vi "HFRR ADV v031 new software.vi"() -> ()   [LabVIEW 2025] (continued)
                        n2406 = Concatenate Strings("Applied Load [grams] :" ("Content"), w3458) -> (w3460:string)
                        n2407 = local read "EVENT LOG"() -> (w3462:string)
                        n2408 = call "Event Log.vi"("Content"=w3460, "EVENT LOG"=w3462) -> ("EVENT LOG"=w3461:string)  [unwired: 8 in, 1 out]
                        n2409 = local write "EVENT LOG"(w3461) -> ()
                      }
                      frame #24 {
                        n2410 = Wait (ms)(milliseconds to wait=u32 50) -> ()  [unwired: 1 out]
                      }
                      frame #25 {
                        n2411 = local read "Set Strk"() -> (w3465:dbl)
                        n2412 = Number To Fractional String(number=w3465, precision (6)=i16 2) -> (F-format string=w3466:string)  [unwired: 2 in]
                        n2413 = Concatenate Strings("Set Stroke [mm] :" ("Content"), w3466) -> (w3468:string)
                        n2414 = local read "EVENT LOG"() -> (w3470:string)
                        n2415 = call "Event Log.vi"("Content"=w3468, "EVENT LOG"=w3470) -> ("EVENT LOG"=w3469:string)  [unwired: 8 in, 1 out]
                        n2416 = local write "EVENT LOG"(w3469) -> ()
                      }
                      frame #26 {
                        n2417 = Wait (ms)(milliseconds to wait=u32 50) -> ()  [unwired: 1 out]
                      }
                      frame #27 {
                        n2418 = local read "Set Temp"() -> (w3473:dbl)
                        n2419 = Number To Fractional String(number=w3473, precision (6)=i16 2) -> (F-format string=w3474:string)  [unwired: 2 in]
                        n2420 = Concatenate Strings("Set Temperature [deg C] :" ("Content"), w3474) -> (w3476:string)
                        n2421 = local read "EVENT LOG"() -> (w3478:string)
                        n2422 = call "Event Log.vi"("Content"=w3476, "EVENT LOG"=w3478) -> ("EVENT LOG"=w3477:string)  [unwired: 8 in, 1 out]
                        n2423 = local write "EVENT LOG"(w3477) -> ()
                      }
                      frame #28 {
                        n2424 = Wait (ms)(milliseconds to wait=u32 50) -> ()  [unwired: 1 out]
                      }
                      frame #29 {
                        n2425 = local read "Set Rh"() -> (w3481:dbl)
                        n2426 = Number To Fractional String(number=w3481, precision (6)=i16 2) -> (F-format string=w3482:string)  [unwired: 2 in]
                        n2427 = Concatenate Strings("Set Humidity [%RH] :" ("Content"), w3482) -> (w3484:string)
                        n2428 = local read "EVENT LOG"() -> (w3486:string)
                        n2429 = call "Event Log.vi"("Content"=w3484, "EVENT LOG"=w3486) -> ("EVENT LOG"=w3485:string)  [unwired: 8 in, 1 out]
                        n2430 = local write "EVENT LOG"(w3485) -> ()
                      }
                      frame #30 {
                        n2431 = Wait (ms)(milliseconds to wait=u32 50) -> ()  [unwired: 1 out]
                      }
                      frame #31 {
                        n2432 = local read "test time"() -> (w3489:dbl)
                        n2433 = Number To Fractional String(number=w3489, precision (6)=i16 1) -> (F-format string=w3490:string)  [unwired: 2 in]
                        n2434 = Concatenate Strings("Test Duration [mins] :" ("Content"), w3490) -> (w3492:string)
                        n2435 = local read "EVENT LOG"() -> (w3494:string)
                        n2436 = call "Event Log.vi"("Content"=w3492, "EVENT LOG"=w3494) -> ("EVENT LOG"=w3493:string)  [unwired: 8 in, 1 out]
                        n2437 = local write "EVENT LOG"(w3493) -> ()
                      }
                      frame #32 {
                        w3495 = dbl[] [] ("History Data")
                        w3496 = cluster{"y":dbl, dbl, "y":dbl}[] [] ("History Data")
                        w3497 = FALSE ("Visible")
                        n2438 = property on="Stroke ( mm )" class="WFChart (strict)"("History Data"=w3496) -> ()  [unwired: 2 in, 2 out]
                        n2439 = property on="Humidity ( %RH )" class="WFChart (strict)"("History Data"=w3495) -> ()  [unwired: 2 in, 2 out]
                        n2440 = property on="Temperature ( Deg C )" class="WFChart (strict)"("History Data"=w3495) -> ()  [unwired: 2 in, 2 out]
                        n2441 = property on="Electrical Contact Resistance ( % )" class="WFChart (strict)"("History Data"=w3495) -> ()  [unwired: 2 in, 2 out]
                        n2442 = property on="Coefficient of Friction" class="WFChart (strict)"("History Data"=w3495) -> ()  [unwired: 2 in, 2 out]
                        n2443 = property on="Frictional Force ( N )" class="WFChart (strict)"("History Data"=w3495) -> ()  [unwired: 2 in, 2 out]
                        n2444 = property on="Coefficient of Friction" class="WFChart (strict)"("History Data"=w3495) -> ()  [unwired: 2 in, 2 out]
                        n2445 = property on="Frictional Force ( N )" class="WFChart (strict)"("History Data"=w3495) -> ()  [unwired: 2 in, 2 out]
                        n2446 = property on="Electrical Contact Resistance ( % )" class="WFChart (strict)"("History Data"=w3495) -> ()  [unwired: 2 in, 2 out]
                        n2447 = property on="Humidity ( %RH )" class="WFChart (strict)"("History Data"=w3495) -> ()  [unwired: 2 in, 2 out]
                        n2448 = property on="Stroke ( mm )" class="WFChart (strict)"("History Data"=w3496) -> ()  [unwired: 2 in, 2 out]
                        n2449 = property on="Temperature ( Deg C )" class="WFChart (strict)"("History Data"=w3495) -> ()  [unwired: 2 in, 2 out]
                        n2450 = property on="Service Password Log" class="Str"("Visible"=w3497) -> ()  [unwired: 2 in, 2 out]
                        n2451 = property on="Password 3" class="Clust (strict)"("Visible"=w3497) -> ()  [unwired: 2 in, 2 out]
                      }
                    }
                    "TEST FILE NAM,E SAVED" <- TRUE ("TEST FILE NAM,E SAVED")
                  }
                }
              }
            }
          }
        }
        n2452 = local write "Test \nStatus"(w2886) -> ()
        n2453 = local write "Save"(w2886) -> ()
        n2454 = local read "Main Tab"() -> (w2880:T2)
        n2455 = case shown="True" w2883 {
          frame False {
            n2456 = local read "Rt 3"() -> (w2955:bool)
            n2457 = case shown="True" w2955 {
              frame False {
              }
              frame True {
                n2458 = local write "Rt 3"(FALSE ("Rt 3")) -> ()
              }
            }
            "Rt" <- TRUE ("Rt")
            "Rt 2" <- FALSE ("Rt")
          }
          frame True {
            n2459 = local read "Rt"() -> (w2961:bool)
            n2460 = local write "Rt 2"(TRUE ("Rt 2")) -> ()
            n2461 = case shown="True" w2961 {
              frame False {
              }
              frame True {
                n2462 = local write "Rt"(FALSE ("Rt")) -> ()
              }
            }
            "Rt 3" <- TRUE ("Rt 3")
          }
        }
        n2463 = case shown="\"Acquire\"" w2880 {
          tunnel: w2882 -> [_ w2989]
          frame Default {
            w2988 = 0.0 ("output")
            n2464 = local write "PID-out"(w2988) -> ()
            n2465 = local write "Frequency ( Hz )"(w2988) -> ()
          }
          frame "Acquire" {
            n2466 = stacked-sequence {
              frame #0 {
                n2467 = local read "Auto Start Test"() -> (w2991:bool)
                n2468 = case shown="True" w2991 {
                  tunnel: "RUN" -> [w3012 w3015]
                  tunnel: [w3012 w3014] -> w2992
                  frame False {
                  }
                  frame True {
                    n2469 = local read "Auto Start Temp"() -> (w3013:bool)
                    n2470 = Or(x=w3015, y=w3013) -> (x .or. y?=w3014:bool)
                  }
                }
                n2471 = local read "clk"() -> (w3011:dbl)
                n2472 = local read "Save"() -> (w3007:bool)
                n2473 = Equal?(x=w3011, y=0.0) -> (x = y?=w3008:bool)
                n2474 = And(x=w3008, y=w3007) -> (x .and. y?=w3009:bool)
                n2475 = Not(x="Engage") -> (.not. x?=w2998:bool)
                n2476 = case shown="False" w2992 {
                  tunnel: [0.0 w3038] -> w2994
                  frame False {
                    (unwired) TRUE ("Visible")
                    n2477 = local read "Auto Start Test"() -> (w3019:bool)
                    n2478 = local write "Start Time"(TRUE ("Start Time")) -> ()
                    n2479 = property on="Stroke 2" class="DigNum (strict)"("Visible"=FALSE) -> ()  [unwired: 2 in, 2 out]
                    n2480 = case shown="False" w3019 {
                      frame False {
                        n2481 = property on="Heater Button" class="Bool (strict)"("DisabledEnum"=T19."Enabled" ("Disabled")) -> ()  [unwired: 2 in, 2 out]
                        n2482 = property on="Humidity" class="Bool (strict)"("DisabledEnum"=T19."Enabled" ("Disabled")) -> ()  [unwired: 2 in, 2 out]
                      }
                      frame True {
                      }
                    }
                    n2483 = case shown="False" "TestCompFlg" {
                      frame False {
                        n2484 = local read "StartFlg"() -> (w3027:bool)
                        n2485 = case shown="True" w3027 {
                          frame False {
                          }
                          frame True {
                            n2486 = stacked-sequence {
                              frame #0 {
                                n2487 = local read "EVENT LOG"() -> (w3031:string)
                                n2488 = call "Event Log.vi"("Content"="Test was interrupted", "EVENT LOG"=w3031) -> ("EVENT LOG"=w3032:string)  [unwired: 8 in, 1 out]
                                n2489 = local write "EVENT LOG"(w3032) -> ()
                                n2490 = property on="RUN" class="Bool (strict)"("Visible"=TRUE) -> ()  [unwired: 2 in, 2 out]
                                n2491 = property on="Auto Start Test" class="Bool (strict)"("Visible"=TRUE) -> ()  [unwired: 2 in, 2 out]
                              }
                              frame #1 {
                                w3034 = FALSE ("StartFlg")
                                n2492 = property on="Heater Button" class="Bool (strict)"("Val(Sgnl)"=FALSE ("Value (Signaling)")) -> ()  [unwired: 2 in, 2 out]
                                n2493 = local write "Heater Button"(w3034) -> ()
                                n2494 = local write "StartFlg"(w3034) -> ()
                                n2495 = local write "Humidity"(w3034) -> ()
                              }
                              frame #2 {
                                n2496 = local write "Due Write"("VC;0" ("Command")) -> ()
                              }
                              frame #3 {
                                n2497 = Wait (ms)(milliseconds to wait=u32 1500) -> ()  [unwired: 1 out]
                              }
                              frame #4 {
                                n2498 = local write "Due Write"("HE;0" ("Command")) -> ()
                              }
                            }
                          }
                        }
                      }
                      frame True {
                      }
                    }
                    n2499 = local write "String 14"("Test will autostart once parameters reach the set value." ("String 14")) -> ()
                  }
                  frame True {
                    (unwired) FALSE ("Visible")
                    n2500 = property on="Stroke 2" class="DigNum (strict)"("Visible"=TRUE) -> ()  [unwired: 2 in, 2 out]
                    n2501 = property on="STOP 2" class="Bool (strict)"("Disabled"=u8 2) -> ()  [unwired: 2 in, 2 out]
                    n2502 = local write "String 14"(" Running....." ("String 14")) -> ()
                    n2503 = property on="Heater Button" class="Bool (strict)"("DisabledEnum"=T19."Disabled and Grayed Out" ("Disabled")) -> ()  [unwired: 2 in, 2 out]
                    n2504 = property on="Humidity" class="Bool (strict)"("DisabledEnum"=T19."Disabled and Grayed Out" ("Disabled")) -> ()  [unwired: 2 in, 2 out]
                    n2505 = case shown="True" "Start Time" {
                      selector: "Start Time" -> [_ w3057]
                      frame False {
                      }
                      frame True {
                        n2506 = Not(x=w3057) -> (.not. x?=w3056:bool)
                        n2507 = local write "Start Time"(w3056) -> ()
                        n2508 = local read "EVENT LOG"() -> (w3058:string)
                        n2509 = call "Event Log.vi"("Content"="Test in progress", "EVENT LOG"=w3058) -> ("EVENT LOG"=w3060:string)  [unwired: 8 in, 1 out]
                        n2510 = local write "EVENT LOG"(w3060) -> ()
                      }
                    }
                    n2511 = disable-structure shown="Enabled" {
                      disable-tunnel: [w3049 w3055] -> w3038
                      frame Disabled {
                        n2512 = local read "Set Hz"() -> (w3052:dbl)
                        n2513 = call <vilib>:"Uniform White Noise Waveform.vi"() -> ("signal out"=w3051:waveform(dbl))  [unwired: 10 in, 1 out]
                        n2514 = Random Number (0-1)() -> (number: 0 to 1=w3048:dbl)
                        n2515 = Add(x=w3052, y=w3051) -> (x+y=w3050:waveform(dbl))
                        n2516 = Multiply(x=ext 0.01 ("y"), y=w3048) -> (x*y=w3046:ext)
                        n2517 = Multiply(x=w3050, y=w3046) -> (x*y=w3049:waveform(ext))
                      }
                      frame Enabled {
                        n2518 = call-poly <vilib>:"Random Number (Range).vi"("lower bound (0)"=49.89, "upper bound (100)"=50.8) -> ("number"=w3055:dbl)  [unwired: 9 in]
                      }
                    }
                    "StartFlg" <- TRUE ("StartFlg")
                  }
                }
                n2519 = case shown="True" w3009 {
                  frame False {
                  }
                  frame True {
                    n2520 = local write "clk"(10.0 ("clk")) -> ()
                    n2521 = Get Date/Time In Seconds() -> (seconds since 1Jan1904=w3063:timestamp)
                    n2522 = To Double Precision Float(number=w3063) -> (double precision float=w3061:dbl)
                    n2523 = local write "acq timer"(w3061) -> ()
                    n2524 = local write "act save time"(w3061) -> ()
                  }
                }
                n2525 = call "Elapsed Time"("Time Target (s)"="Countdown", "Reset"=w2998) -> ("Elapsed Time (s)"=w3003:dbl, "Time has Elapsed"=w3001:bool)  [unwired: 10 in, 6 out]
                "Countdown 2" <- w3003
                n2526 = Subtract(x=w3003, y=2.0) -> (x-y=w3006:dbl)
                n2527 = Less?(x=w3006, y="Countdown") -> (x < y?=w3004:bool)
                n2528 = And(x=w3004, y=w3001) -> (x .and. y?=w3000:bool)
                n2529 = case shown="True" w3000 {
                  frame False {
                  }
                  frame True {
                    (unwired) dbl[] [] ("History Data")
                    n2530 = local write "Engage"(FALSE ("Engage")) -> ()
                    n2531 = local write "RUN"(TRUE ("RUN")) -> ()
                    n2532 = local read "Humidity ( %RH )"() -> (→"Rh Before":dbl)
                  }
                }
                n2533 = local read "Test \nStatus"() -> (w2996:bool)
                n2534 = Select(t=w2994, s=w2996, f=0.0) -> (s? t:f=w2995:dbl)
                n2535 = local write "Frequency ( Hz )"(w2995) -> ()
              }
              frame #1 {
                w3086 = 1000000.0 ("x")
                # "HC;1/0\nST;VALUE"
                # "Elapsed time\ncof\nstroke\nAir temp\nTemp\nHumidity"
                # "acq timer\n\nact save time"
                # "convert to microseconds"
                n2536 = local read "COUNT"() -> (w3069:i32)
                n2537 = local read "Rate"() -> (w3082:dbl)
                n2538 = Divide(x=w3086, y=w3082) -> (x/y=w3087:dbl)
                n2539 = Greater Or Equal?(x=w3069, y=250) -> (x >= y?=w3068:bool)
                n2540 = Get Date/Time In Seconds() -> (seconds since 1Jan1904=w3089:timestamp)
                n2541 = case shown="True" w3068 {
                  frame False {
                    n2542 = local read "COUNT"() -> (w3090:i32)
                    n2543 = Increment(x=w3090) -> (x+1=w3091:i32)
                    n2544 = local write "COUNT"(w3091) -> ()
                  }
                  frame True {
                    n2545 = local write "COUNT"(0 ("COUNT")) -> ()
                  }
                }
                n2546 = local read "Samplingtime 2"() -> (w3067:dbl)
                n2547 = local read "act save time"() -> (w3084:dbl)
                n2548 = Divide(x=w3087, y=w3086) -> (x/y=w3085:dbl)
                n2549 = To Double Precision Float(number=w3089) -> (double precision float=w3078:dbl)
                n2550 = Add(x=w3084, y=w3067) -> (x+y=w3083:dbl)
                n2551 = local read "acq timer"() -> (w3088:dbl)
                n2552 = local read "COUNT"() -> (w3071:i32)
                n2553 = Greater Or Equal?(x=w3078, y=w3083) -> (x >= y?=w3066:bool)
                n2554 = Multiply(x=w3085, y=w3071) -> (x*y=w3077:dbl)
                n2555 = Subtract(x=w3078, y=w3088) -> (x-y=w3080:dbl)
                n2556 = local read "Save"() -> (w3081:bool)
                n2557 = Add(x=w3080, y=w3077) -> (x+y=w3064:dbl)
                "Elapsed time 3" <- w3064
                n2558 = And(x=w3066, y=w3081) -> (x .and. y?=w3079:bool)
                n2559 = Divide(x=w3064, y=60.0) -> (x/y=w3075:dbl)
                n2560 = local read "Test \nStatus"() -> (w3065:bool)
                n2561 = local read "clk"() -> (w3072:dbl)
                n2562 = Equal?(x=w3072, y=10.0) -> (x = y?=w3074:bool)
                n2563 = case shown="True" w3079 {
                  tunnel: w3078 -> [_ w3203]
                  tunnel: [FALSE ("Boolean 2") TRUE ("Boolean 2")] -> _
                  frame False {
                  }
                  frame True {
                    w3157 = ";" ("Substring")
                    # "Pid out/\nFreq response value"
                    n2564 = local write "act save time"(w3203) -> ()
                    n2565 = local read "FILE"() -> (w3151:string)
                    n2566 = call "file check.vi"("file name in"=w3151) -> ("error out"=w3154:errorcluster, "file name out"=w3149:string)  [unwired: 9 in]
                    n2567 = local read "LVDT STROKE"() -> (w3146:dbl)
                    n2568 = local read "Add up Stroke"() -> (w3144:dbl)
                    n2569 = call "FILE PATH CREATION.vi"("error in"=w3154, "FILE NAME :"=w3149) -> ("FILE OUT"=w3152:path)  [unwired: 8 in, 1 out]
                    n2570 = Concatenate Strings(w3149, ".dgf" ("Substring")) -> (w3153:string)
                    n2571 = Subtract(x=w3146, y=w3144) -> (x-y=w3145:dbl)
                    n2572 = Absolute Value(x=w3145) -> (abs(x)=w3143:dbl)
                    n2573 = local read "FF 2"() -> (→"Frictional Force ( N )" →"Frictional Force ( N )":dbl)
                    n2574 = Build Path(base path=w3152, name or relative path=w3153) -> (appended path=w3148:path)
                    n2575 = local read "COF 2"() -> (w3162:dbl)
                    "Coefficient of Friction" <- w3162
                    "COF 4" <- w3162
                    "Coefficient of Friction" <- w3162
                    n2576 = local read "TEMP"() -> (w3165:dbl)
                    "Temperature ( Deg C )" <- w3165
                    n2577 = local read "Humidity ( %RH )"() -> (w3164:dbl)
                    "Humidity ( %RH )" <- w3164
                    "Humidity ( %RH )" <- w3164
                    n2578 = local read "Frequency ( Hz )"() -> (w3171:dbl)
                    n2579 = local read "LVDT STROKE DISPLAY"() -> (w3140:dbl)
                    n2580 = call <vilib>:"Mean PtByPt.vi"("x"=w3143, "sample length"="STROKE FILTER") -> ("mean"=→"LVDT STROKE Actual":dbl)  [unwired: 2 in, 1 out]
                    n2581 = local read "Elapsed time"() -> (w3196:dbl)
                    n2582 = local read "AIR TEMP"() -> (w3169:dbl)
                    n2583 = local read "PID-out"() -> (w3174:dbl)
                    n2584 = local write "Temperature ( Deg C )"(w3165) -> ()
                    n2585 = Number To Fractional String(number=w3140, width (-)=i16 9 ("precision (6)"), precision (6)=i16 6) -> (F-format string=w3189:string)  [unwired: 1 in]
                    n2586 = Number To Fractional String(number=w3169, width (-)=i16 9 ("precision (6)"), precision (6)=i16 3) -> (F-format string=w3188:string)  [unwired: 1 in]
                    n2587 = Number To Fractional String(number=w3165, width (-)=i16 9 ("precision (6)"), precision (6)=i16 3) -> (F-format string=w3185:string)  [unwired: 1 in]
                    n2588 = Number To Fractional String(number=w3164, width (-)=i16 9 ("precision (6)"), precision (6)=i16 3) -> (F-format string=w3182:string)  [unwired: 1 in]
                    n2589 = Number To Fractional String(number=0.0, width (-)=i16 9 ("precision (6)"), precision (6)=i16 3) -> (F-format string=w3179:string)  [unwired: 1 in]
                    n2590 = Number To Fractional String(number=w3174, width (-)=i16 9 ("precision (6)"), precision (6)=i16 3) -> (F-format string=w3175:string)  [unwired: 1 in]
                    n2591 = Number To Fractional String(number=w3171, width (-)=i16 9 ("precision (6)"), precision (6)=i16 3) -> (F-format string=w3170:string)  [unwired: 1 in]
                    n2592 = Number To Fractional String(number=w3162, width (-)=i16 9 ("precision (6)"), precision (6)=i16 6) -> (F-format string=w3197:string)  [unwired: 1 in]
                    n2593 = Number To Fractional String(number=w3196, width (-)=i16 14 ("precision (6)"), precision (6)=i16 3) -> (F-format string=w3198:string)  [unwired: 1 in]
                    n2594 = Bundle("y"=1.02, "LVDT STROKE DISPLAY"=w3140, "y"=0.98) -> (w3163:T30)  [unwired: 1 in]
                    n2595 = Number To Fractional String(number="Ambient Humidity :", width (-)=i16 9 ("precision (6)"), precision (6)=i16 6) -> (F-format string=w3155:string)  [unwired: 1 in]
                    n2596 = local read "RUN"() -> (w3161:bool)
                    n2597 = case shown="True" w3161 {
                      tunnel: w3163 -> [_ w3208]
                      tunnel: w3140 -> [_ w3207]
                      tunnel: w3140 -> [_ w3205]
                      tunnel: w3140 -> [_ w3206]
                      frame False {
                      }
                      frame True {
                        "Stroke ( mm )" <- w3208
                        "Stroke ( mm )" <- w3208
                        "Stroke 4" <- w3207
                        "Stroke 3" <- w3205
                        "Stroke 2" <- w3206
                        "measured_stroke" <- w3205
                      }
                    }
                    n2598 = Concatenate Strings(w3198, w3157, w3197, w3157, w3189, w3157, w3188, w3157, w3185, w3157, w3182, w3157, w3179, w3157, w3175, w3157, w3170, w3157, w3155, "\r") -> (w3195:string)
                    n2599 = call <vilib>:"Write Characters To File.vi"("append to file? (new file:F)"=TRUE, "character string"=w3195, "file path (dialog if empty)"=w3148) -> ()  [unwired: 2 in, 1 out]
                    "refresh flag" <- TRUE ("refresh flag")
                  }
                }
                n2600 = case shown="True" w3065 {
                  tunnel: w3075 -> [_ w3101]
                  tunnel: w3080 -> [_ w3111]
                  tunnel: [0.0 w3107] -> _
                  tunnel: w3074 -> [_ w3106]
                  tunnel: [0.0 w3105] -> _
                  tunnel: w3064 -> [_ w3105]
                  tunnel: w3078 -> [w3094 _]
                  frame False {
                    n2601 = local write "acq timer"(w3094) -> ()
                    n2602 = local write "Test Duration Status"(0.0 ("Test Duration Status")) -> ()
                  }
                  frame True {
                    n2603 = local read "Set Hz"() -> (w3108:dbl)
                    n2604 = local write "Elapsed time"(w3101) -> ()
                    n2605 = local read "test time"() -> (w3100:dbl)
                    n2606 = Multiply(x=w3111, y=w3108) -> (x*y=w3110:dbl)
                    n2607 = case shown="False" w3106 {
                      tunnel: w3110 -> [w3112 _]
                      tunnel: [w3112 1.0] -> w3107
                      frame False {
                        n2608 = local write "Cycles elapsed"(w3112) -> ()
                      }
                      frame True {
                      }
                    }
                    n2609 = Greater?(x=w3101, y=w3100) -> (0:w3109:bool)
                    n2610 = Subtract(x=w3100, y=w3101) -> (x-y=w3099:dbl)
                    n2611 = Multiply(x=w3099, y=60.0) -> (x*y=w3098:dbl)
                    n2612 = local write "Time Remaining"(w3098) -> ()
                    n2613 = local write "Remaining Time"(w3098) -> ()
                    n2614 = case shown="True" w3109 {
                      frame False {
                      }
                      frame True {
                        n2615 = stacked-sequence {
                          frame #0 {
                            w3117 = T19."Enabled" ("Disabled")
                            w3116 = FALSE ("TEST FILE NAM,E SAVED")
                            w3118 = "" ("FILE")
                            w3119 = TRUE ("Visible")
                            n2616 = local write "Humidity"(FALSE ("Humidity")) -> ()
                            n2617 = local write "RUN"(FALSE ("OK Button 2")) -> ()
                            n2618 = local write "Heater Button"(FALSE ("Heater Button")) -> ()
                            n2619 = local write "Auto Start Test"(FALSE ("Auto Start Test")) -> ()
                            n2620 = local write "TestCompFlg"(TRUE ("StpFlg")) -> ()
                            n2621 = local read "Humidity ( %RH )"() -> (→"Rh After":dbl)
                            n2622 = property on="STOP 2" class="Bool (strict)"("Disabled"=u8 0) -> ()  [unwired: 2 in, 2 out]
                            n2623 = local read "EVENT LOG"() -> (w3124:string)
                            n2624 = call "Event Log.vi"("Content"="Test Completed", "EVENT LOG"=w3124) -> ("EVENT LOG"=w3123:string)  [unwired: 8 in, 1 out]
                            n2625 = property on="RUN" class="Bool (strict)"("Visible"=w3119) -> ()  [unwired: 2 in, 2 out]
                            n2626 = property on="Auto Start Test" class="Bool (strict)"("Visible"=w3119) -> ()  [unwired: 2 in, 2 out]
                            n2627 = local write "Batch Ref Num :"(w3118) -> ()
                            n2628 = local write "FILE"(w3118) -> ()
                            n2629 = local write "EVENT LOG"(w3123) -> ()
                            n2630 = local write "TEST FILE NAM,E SAVED"(w3116) -> ()
                            n2631 = local write "Fuel Discription :"(w3118) -> ()
                            n2632 = local write "START TEMP"(w3116) -> ()
                            n2633 = local write "Remarks :"(w3118) -> ()
                            n2634 = local write "Main Dashboard Buttons"(T1."Imaging" ("Main Dashboard Buttons")) -> ()
                            n2635 = local write "Main Tab"(T2."Adv Scar" ("Main Tab")) -> ()
                            n2636 = property on="FRICVALZ 2" class="Bool (strict)"("DisabledEnum"=w3117) -> ()  [unwired: 2 in, 2 out]
                            n2637 = property on="FRICVALZ 3" class="Bool (strict)"("DisabledEnum"=w3117) -> ()  [unwired: 2 in, 2 out]
                            n2638 = property on="FRICVALZ 4" class="Bool (strict)"("DisabledEnum"=w3117) -> ()  [unwired: 2 in, 2 out]
                          }
                          frame #1 {
                            n2639 = Wait (ms)(milliseconds to wait=u32 1500) -> ()  [unwired: 1 out]
                          }
                          frame #2 {
                            n2640 = local write "Due Write"("VC;0") -> ()
                          }
                          frame #3 {
                            n2641 = Wait (ms)(milliseconds to wait=u32 1500) -> ()  [unwired: 1 out]
                          }
                          frame #4 {
                            n2642 = local write "Due Write"("VC;0") -> ()
                          }
                          frame #5 {
                            n2643 = Wait (ms)(milliseconds to wait=u32 1500) -> ()  [unwired: 1 out]
                          }
                          frame #6 {
                            n2644 = local write "Due Write"("ST;0") -> ()
                          }
                          frame #7 {
                            n2645 = local write "measured_stroke"(0.0 ("measured_stroke")) -> ()
                            n2646 = Wait (ms)(milliseconds to wait=u32 1500) -> ()  [unwired: 1 out]
                          }
                          frame #8 {
                            n2647 = local write "Due Write"("HE;0") -> ()
                          }
                        }
                      }
                    }
                    n2648 = Divide(x=w3101, y=w3100) -> (x/y=w3104:dbl)
                    n2649 = Multiply(x=w3104, y=100.0) -> (x*y=w3102:dbl)
                    n2650 = local write "Test Duration Status"(w3102) -> ()
                  }
                }
              }
              frame #2 {
                n2651 = case shown="True" "Heater Button" {
                  tunnel: [0.0 ("output") w3231] -> w3209
                  frame False {
                    w3212 = TRUE ("tmpchk")
                    n2652 = local read "TEMP"() -> (w3213:dbl)
                    n2653 = local write "Temp ini"(w3213) -> ()
                    n2654 = local write "Reset 4"(w3212) -> ()
                    n2655 = local write "tmpchk"(w3212) -> ()
                    n2656 = local write "reinit"(TRUE ("reinit")) -> ()
                    n2657 = local write "manual temp log"(TRUE ("manual temp log")) -> ()
                  }
                  frame True {
                    # "Logic to turn off\nthe heater when \ntemp is not rising.\nTime - 60 sec\nDelta t- 5°c"
                    n2658 = local read "Temp ini"() -> (w3220:dbl)
                    n2659 = local read "Auto Start Test"() -> (w3216:bool)
                    n2660 = Less?(x=w3220, y=53.0) -> (x < y?=w3218:bool)
                    n2661 = case shown="False" w3216 {
                      frame False {
                        n2662 = local read "Set Temp"() -> (w3240:dbl)
                        n2663 = local read "TEMP"() -> (w3239:dbl)
                        n2664 = Subtract(x=w3240, y=w3239) -> (x-y=w3238:dbl)
                        n2665 = Absolute Value(x=w3238) -> (abs(x)=w3237:dbl)
                        n2666 = Less?(x=w3237, y=0.5) -> (x < y?=w3235:bool)
                        n2667 = case shown="True" w3235 {
                          tunnel: "manual temp log" -> [_ w3241]
                          frame False {
                          }
                          frame True {
                            n2668 = case shown="True" w3241 {
                              selector: w3241 -> [_ w3242]
                              frame False {
                              }
                              frame True {
                                # "#Event log"
                                n2669 = Not(x=w3242) -> (.not. x?=w3243:bool)
                                n2670 = local write "manual temp log"(w3243) -> ()
                                n2671 = local read "EVENT LOG"() -> (w3246:string)
                                n2672 = call "Event Log.vi"("Content"="Target Temperature reached", "EVENT LOG"=w3246) -> ("EVENT LOG"=w3245:string)  [unwired: 8 in, 1 out]
                                n2673 = local write "EVENT LOG"(w3245) -> ()
                              }
                            }
                          }
                        }
                      }
                      frame True {
                        n2674 = local write "manual temp log"(TRUE ("manual temp log")) -> ()
                      }
                    }
                    n2675 = And(x="tmpchk", y=w3218) -> (x .and. y?=w3221:bool)
                    n2676 = case shown="True" w3221 {
                      frame False {
                      }
                      frame True {
                        n2677 = call "Elapsed Time8"("Time Target (s)"=300.0, "Reset"="Reset 4") -> ("Time has Elapsed"=w3248:bool)  [unwired: 10 in, 7 out]
                        n2678 = flat-sequence {
                          tunnel: w3248 -> [_]
                          frame #0 {
                            n2679 = local write "Reset 4"(FALSE ("Reset 4")) -> ()
                          }
                        }
                        n2680 = case shown="True" w3248 {
                          frame False {
                          }
                          frame True {
                            n2681 = local read "Temp ini"() -> (w3255:dbl)
                            n2682 = Add(x=w3255, y=5.0) -> (x+y=w3253:dbl)
                            n2683 = local read "TEMP"() -> (w3256:dbl)
                            n2684 = Greater?(x=w3256, y=w3253) -> (0:w3254:bool)
                            n2685 = case shown="False" w3254 {
                              frame False {
                                n2686 = local write "Heater Button"(FALSE ("Heater Button")) -> ()
                              }
                              frame True {
                                n2687 = local write "tmpchk"(FALSE ("tmpchk")) -> ()
                              }
                            }
                          }
                        }
                      }
                    }
                    n2688 = local read "Set Temp"() -> (w3229:dbl)
                    n2689 = local read "TEMP"() -> (w3223:dbl)
                    n2690 = call-poly <vilib>:"PID.vi"("reinitialize? (F)"="reinit", "dt (s)"=-1.0, "process variable"=w3223, "setpoint"=w3229) -> ("output"=w3226:dbl)  [unwired: 6 in, 1 out]
                    n2691 = Subtract(x=w3229, y=w3223) -> (x-y=w3230:dbl)
                    n2692 = Add(x=w3229, y=0.5) -> (x+y=w3227:dbl)
                    n2693 = Greater Or Equal?(x=w3223, y=w3227) -> ()  [unwired: 1 out]
                    n2694 = Select(t=0.0, s=FALSE, f=w3226) -> (s? t:f=w3225:dbl)
                    "PID output" <- w3225
                    n2695 = flat-sequence {
                      tunnel: w3225 -> [w3259]
                      tunnel: [w3259] -> w3231
                      frame #0 {
                        n2696 = local write "reinit"(FALSE ("reinit")) -> ()
                      }
                    }
                    n2697 = Bundle(w3230, "output"=w3225, "TEMP"=w3223) -> ()  [unwired: 1 in, 1 out]
                  }
                }
                "PID-out" <- w3209
              }
              frame #3 {
                n2698 = local read "TEMP"() -> (w3261:dbl)
                n2699 = Greater Or Equal?(x=w3261, y="Set Temp 2") -> (x >= y?=w3266:bool)
                n2700 = case shown="True" w3266 {
                  tunnel: [FALSE TRUE] -> w3264
                  frame False {
                  }
                  frame True {
                  }
                }
                "Status 13" <- w3264
                n2701 = And(x=w3264, y="trip1 8") -> (x .and. y?=w3263:bool)
                n2702 = case shown="True" w3263 {
                  frame False {
                    n2703 = local write "Heater Trip Temp"(TRUE ("Heater Trip Temp")) -> ()
                  }
                  frame True {
                    w3269 = FALSE ("OK Button 2")
                    n2704 = case shown="True" "Heater Trip Temp" {
                      selector: "Heater Trip Temp" -> [_ w3271]
                      frame False {
                      }
                      frame True {
                        n2705 = Not(x=w3271) -> (.not. x?=w3270:bool)
                        n2706 = local read "EVENT LOG"() -> (w3274:string)
                        n2707 = local write "Heater Trip Temp"(w3270) -> ()
                        n2708 = call "Event Log.vi"("Content"="Heater Trip", "EVENT LOG"=w3274) -> ("EVENT LOG"=w3273:string)  [unwired: 8 in, 1 out]
                        n2709 = local write "EVENT LOG"(w3273) -> ()
                      }
                    }
                    n2710 = local write "RUN"(w3269) -> ()
                    n2711 = property on="Auto Start Test" class="Bool (strict)"("Value"=w3269) -> ()  [unwired: 2 in, 2 out]
                    n2712 = local write "Heater Button"(w3269) -> ()
                  }
                }
              }
            }
            n2713 = case shown="False" w2989 {
              frame False {
                n2714 = disable-structure shown="Disabled" {
                  frame Disabled {
                    n2715 = stacked-sequence {
                      frame #0 {
                        n2716 = local write "RUN"(FALSE ("OK Button 2")) -> ()
                      }
                      frame #1 {
                      }
                    }
                  }
                  frame Enabled {
                  }
                }
              }
              frame True {
              }
            }
          }
        }
        n2717 = local read "Reset Graph"() -> (w2879:bool)
        n2718 = case shown="True" w2879 {
          selector: w2879 -> [_ w2896]
          frame False {
          }
          frame True {
            w2910 = 0.0 ("X Scale.Range:Maximum")
            n2719 = Not(x=w2896) -> (.not. x?=w2895:bool)
            n2720 = local write "Reset Graph"(w2895) -> ()
            n2721 = property on="Electrical Contact Resistance ( % )" class="WFChart (strict)"("XScale.Maximum"=600.0 ("X Scale.Range:Maximum"), "XScale.Minimum"=0.0 ("X Scale.Range:Minimum"), "YScale.Maximum"=100.0 ("Y Scale.Range:Maximum"), "YScale.Minimum"=0.0 ("Y Scale.Range:Minimum")) -> ()  [unwired: 2 in, 2 out]
            n2722 = property on="Frictional Force ( N )" class="WFChart (strict)"("XScale.Maximum"=600.0 ("X Scale.Range:Maximum"), "XScale.Minimum"=0.0 ("X Scale.Range:Minimum"), "YScale.Maximum"=100.0 ("Y Scale.Range:Maximum"), "YScale.Minimum"=0.0 ("Y Scale.Range:Minimum")) -> ()  [unwired: 2 in, 2 out]
            n2723 = property on="Temperature ( Deg C )" class="WFChart (strict)"("XScale.Maximum"=600.0 ("X Scale.Range:Maximum"), "XScale.Minimum"=0.0 ("X Scale.Range:Minimum"), "YScale.Maximum"=100.0 ("Y Scale.Range:Maximum"), "YScale.Minimum"=0.0 ("Y Scale.Range:Minimum")) -> ()  [unwired: 2 in, 2 out]
            n2724 = property on="Humidity ( %RH )" class="WFChart (strict)"("XScale.Maximum"=600.0 ("X Scale.Range:Maximum"), "XScale.Minimum"=0.0 ("X Scale.Range:Minimum"), "YScale.Maximum"=100.0 ("Y Scale.Range:Maximum"), "YScale.Minimum"=0.0 ("Y Scale.Range:Minimum")) -> ()  [unwired: 2 in, 2 out]
            n2725 = property on="Stroke ( mm )" class="WFChart (strict)"("XScale.Maximum"=600.0 ("X Scale.Range:Maximum"), "XScale.Minimum"=0.0 ("X Scale.Range:Minimum"), "YScale.Maximum"=100.0 ("Y Scale.Range:Maximum"), "YScale.Minimum"=0.0 ("Y Scale.Range:Minimum")) -> ()  [unwired: 2 in, 2 out]
            n2726 = property on="Coefficient of Friction" class="WFChart (strict)"("XScale.Maximum"=600.0 ("X Scale.Range:Maximum"), "XScale.Minimum"=0.0 ("X Scale.Range:Minimum"), "YScale.Maximum"=100.0 ("Y Scale.Range:Maximum"), "YScale.Minimum"=0.0 ("Y Scale.Range:Minimum")) -> ()  [unwired: 2 in, 2 out]
            n2727 = property on="Electrical Contact Resistance ( % )" class="WFChart (strict)"("XScale.Minimum"=0.0 ("X Scale.Range:Minimum"), "XScale.Maximum"=600.0 ("X Scale.Range:Maximum"), "YScale.Minimum"=0.0 ("Y Scale.Range:Minimum"), "YScale.Maximum"=100.0 ("Y Scale.Range:Maximum")) -> ()  [unwired: 2 in, 2 out]
            n2728 = property on="Temperature ( Deg C )" class="WFChart (strict)"("XScale.Minimum"=0.0 ("X Scale.Range:Minimum"), "XScale.Maximum"=600.0 ("X Scale.Range:Maximum"), "YScale.Minimum"=0.0 ("Y Scale.Range:Minimum"), "YScale.Maximum"=100.0 ("Y Scale.Range:Maximum")) -> ()  [unwired: 2 in, 2 out]
            n2729 = property on="Coefficient of Friction" class="WFChart (strict)"("XScale.Minimum"=0.0 ("X Scale.Range:Minimum"), "XScale.Maximum"=600.0 ("X Scale.Range:Maximum"), "YScale.Maximum"=1.0 ("X Scale.Range:Minimum"), "YScale.Minimum"=0.0 ("X Scale.Range:Minimum")) -> ()  [unwired: 2 in, 2 out]
            n2730 = property on="Frictional Force ( N )" class="WFChart (strict)"("XScale.Maximum"=600.0 ("X Scale.Range:Maximum"), "XScale.Minimum"=w2910, "YScale.Maximum"=10.0 ("Y Scale.Range:Maximum"), "YScale.Minimum"=w2910) -> ()  [unwired: 2 in, 2 out]
            n2731 = property on="Stroke ( mm )" class="WFChart (strict)"("XScale.Maximum"=600.0 ("X Scale.Range:Maximum"), "XScale.Minimum"=0.0 ("X Scale.Range:Minimum"), "YScale.Maximum"=100.0 ("Y Scale.Range:Maximum"), "YScale.Minimum"=0.0 ("Y Scale.Range:Minimum")) -> ()  [unwired: 2 in, 2 out]
            n2732 = property on="Humidity ( %RH )" class="WFChart (strict)"("XScale.Maximum"=600.0 ("X Scale.Range:Maximum"), "XScale.Minimum"=0.0 ("X Scale.Range:Minimum"), "YScale.Maximum"=100.0 ("Y Scale.Range:Maximum"), "YScale.Minimum"=0.0 ("Y Scale.Range:Minimum")) -> ()  [unwired: 2 in, 2 out]
          }
        }
      }
      frame "Compare Files" {
        # "Elapsed time\ncof\nstroke\nAir temp\nTemp\nHumidity"
        n2733 = case shown="True" "RSTV1 2" {
          frame False {
          }
          frame True {
            n2734 = property on="Humidity ( %RH )" class="XYGraph (strict)"("Y Scale.Display Format:Precision"=u8 0 ("Y Scale.Format & Precision:Precision")) -> ()  [unwired: 2 in, 2 out]
            n2735 = property on="Humidity ( %RH )" class="XYGraph (strict)"("X Scale.Range:Minimum"=0.0, "X Scale.Range:Maximum"=75.0, "Y Scale.Range:Minimum"=48.0, "Y Scale.Range:Maximum"=58.0) -> ()  [unwired: 2 in, 2 out]
          }
        }
        n2736 = case shown="True" "RST CP 2" {
          frame False {
          }
          frame True {
            n2737 = property on="XY Graph 13" class="XYGraph (strict)"("Y Scale.Display Format:Precision"=u8 0 ("Y Scale.Format & Precision:Precision")) -> ()  [unwired: 2 in, 2 out]
            n2738 = property on="XY Graph 13" class="XYGraph (strict)"("X Scale.Range:Minimum"=0.0, "X Scale.Range:Maximum"=75.0, "Y Scale.Range:Minimum"=0.0, "Y Scale.Range:Maximum"=100.0) -> ()  [unwired: 2 in, 2 out]
          }
        }
        n2739 = case shown="True" "RST CP" {
          frame False {
          }
          frame True {
            n2740 = property on="Sample Temperature ( °C )" class="XYGraph (strict)"("Y Scale.Display Format:Precision"=u8 2 ("Y Scale.Format & Precision:Precision")) -> ()  [unwired: 2 in, 2 out]
            n2741 = property on="Sample Temperature ( °C )" class="XYGraph (strict)"("X Scale.Range:Minimum"=0.0, "X Scale.Range:Maximum"=75.0, "Y Scale.Range:Minimum"=58.0, "Y Scale.Range:Maximum"=62.0) -> ()  [unwired: 2 in, 2 out]
          }
        }
        n2742 = case shown="True" "RSTV1 3" {
          frame False {
          }
          frame True {
            n2743 = property on="Air Temperature  ( °C )" class="XYGraph (strict)"("Y Scale.Display Format:Precision"=u8 2 ("Y Scale.Format & Precision:Precision")) -> ()  [unwired: 2 in, 2 out]
            n2744 = property on="Air Temperature  ( °C )" class="XYGraph (strict)"("X Scale.Range:Minimum"=0.0 ("Y Scale.Range:Minimum"), "X Scale.Range:Maximum"=75.0 ("Y Scale.Range:Maximum"), "Y Scale.Range:Minimum"=20.0 ("X Scale.Range:Minimum"), "Y Scale.Range:Maximum"=26.0 ("X Scale.Range:Maximum")) -> ()  [unwired: 2 in, 2 out]
          }
        }
        n2745 = case shown="True" "RSTV1 4" {
          frame False {
          }
          frame True {
            n2746 = property on="Stroke ( mm )" class="XYGraph (strict)"("Y Scale.Display Format:Precision"=u8 2 ("Y Scale.Format & Precision:Precision")) -> ()  [unwired: 2 in, 2 out]
            n2747 = property on="Stroke ( mm )" class="XYGraph (strict)"("X Scale.Range:Minimum"=0.0 ("Y Scale.Range:Maximum"), "X Scale.Range:Maximum"=75.0 ("X Scale.Range:Minimum"), "Y Scale.Range:Minimum"=0.98, "Y Scale.Range:Maximum"=1.02) -> ()  [unwired: 2 in, 2 out]
          }
        }
        n2748 = case shown="True" "rstv2" {
          frame False {
          }
          frame True {
            n2749 = property on="Coefficient Of Friction" class="XYGraph (strict)"("Y Scale.Display Format:Precision"=u8 3 ("Y Scale.Format & Precision:Precision")) -> ()  [unwired: 2 in, 2 out]
            n2750 = property on="Coefficient Of Friction" class="XYGraph (strict)"("X Scale.Range:Minimum"=0.0 ("Y Scale.Range:Maximum"), "X Scale.Range:Maximum"=75.0, "Y Scale.Range:Minimum"=0.0, "Y Scale.Range:Maximum"=1.0 ("X Scale.Range:Minimum")) -> ()  [unwired: 2 in, 2 out]
          }
        }
        n2751 = case shown="True" "RST CP 3" {
          frame False {
          }
          frame True {
            n2752 = property on="Air Temp ( °C ) vs Humidity ( % RH )" class="XYGraph (strict)"("X Scale.Range:Minimum"=18.0, "X Scale.Range:Maximum"=28.0 ("X Scale.Range:Minimum"), "Y Scale.Range:Minimum"=30.0 ("X Scale.Range:Minimum"), "Y Scale.Range:Maximum"=70.0 ("X Scale.Range:Minimum")) -> ()  [unwired: 2 in, 2 out]
          }
        }
        n2753 = case shown="True" "OPEN 1" {
          frame False {
          }
          frame True {
            (unwired) 0  # existing file
            w3550 = "Choose a datalog file to open"  # prompt
            n2754 = local write "OPEN 1"(FALSE ("OPEN 1")) -> ()
            n2755 = String To Path(string="C:\\LAB-IQ\\Data\\") -> (path=w3535:path)
            n2756 = File Dialog(6:"*.dgf" ("pattern"), 7:w3550, 11:w3535) -> (0:w3533:errorcluster, 3:w3541:path)  [unwired: 4 in, 2 out]
            n2757 = Unbundle(w3533) -> ()  [unwired: 3 out]
            n2758 = Strip Path(path=w3541) -> (name=w3540:string)  [unwired: 1 out]
            n2759 = Path To String(path=w3541) -> (string=w3536:string)
            "string1" <- w3536
            n2760 = Match Pattern(string=w3540, regular expression=".dgf") -> (before substring=→"String Control":string)  [unwired: 1 in, 3 out]
            n2761 = Match Pattern(string=w3536, regular expression=".dgf" ("substring (\"\")")) -> (before substring=w3546:string)  [unwired: 1 in, 3 out]
            n2762 = Concatenate Strings(w3546, ".duf" ("Substring")) -> (w3542:string)
            n2763 = String To Path(string=w3542) -> (path=w3547:path)
            n2764 = call <vilib>:"Read Characters From File.vi"("file path (dialog if empty)"=w3547, "start of read offset (chars.:0)"=60 ("start of read offset (chars.: 0)")) -> ("character string"=→"String Control 2":string)  [unwired: 4 in, 3 out]
          }
        }
        n2765 = case shown="True" "OPEN 2" {
          frame False {
          }
          frame True {
            (unwired) 0  # existing file
            w3568 = "Choose a datalog file to open"  # prompt
            n2766 = local write "OPEN 2"(FALSE ("OPEN 1")) -> ()
            n2767 = String To Path(string="C:\\LAB-IQ\\Data\\") -> (path=w3553:path)
            n2768 = File Dialog(6:"*.dgf" ("pattern"), 7:w3568, 11:w3553) -> (0:w3551:errorcluster, 3:w3559:path)  [unwired: 4 in, 2 out]
            n2769 = Unbundle(w3551) -> ()  [unwired: 3 out]
            n2770 = Strip Path(path=w3559) -> (name=w3557:string)  [unwired: 1 out]
            n2771 = Path To String(path=w3559) -> (string=w3554:string)
            "string1 2" <- w3554
            n2772 = Match Pattern(string=w3557, regular expression=".dgf") -> (before substring=→"String Control 3":string)  [unwired: 1 in, 3 out]
            n2773 = Match Pattern(string=w3554, regular expression=".dgf" ("substring (\"\")")) -> (before substring=w3565:string)  [unwired: 1 in, 3 out]
            n2774 = Concatenate Strings(w3565, ".duf" ("Substring")) -> (w3562:string)
            n2775 = String To Path(string=w3562) -> (path=w3560:path)
            n2776 = call <vilib>:"Read Characters From File.vi"("file path (dialog if empty)"=w3560, "start of read offset (chars.:0)"=60 ("start of read offset (chars.: 0)")) -> ("character string"=→"String Control 4":string)  [unwired: 4 in, 3 out]
          }
        }
        n2777 = case shown="True" "OPEN 3" {
          frame False {
          }
          frame True {
            (unwired) 0  # existing file
            w3586 = "Choose a datalog file to open"  # prompt
            n2778 = local write "OPEN 3"(FALSE ("OPEN 1")) -> ()
            n2779 = String To Path(string="C:\\LAB-IQ\\Data\\") -> (path=w3571:path)
            n2780 = File Dialog(6:"*.dgf" ("pattern"), 7:w3586, 11:w3571) -> (0:w3569:errorcluster, 3:w3577:path)  [unwired: 4 in, 2 out]
            n2781 = Unbundle(w3569) -> ()  [unwired: 3 out]
            n2782 = Strip Path(path=w3577) -> (name=w3575:string)  [unwired: 1 out]
            n2783 = Path To String(path=w3577) -> (string=w3572:string)
            "string1 3" <- w3572
            n2784 = Match Pattern(string=w3575, regular expression=".dgf") -> (before substring=→"String Control 5":string)  [unwired: 1 in, 3 out]
            n2785 = Match Pattern(string=w3572, regular expression=".dgf" ("substring (\"\")")) -> (before substring=w3582:string)  [unwired: 1 in, 3 out]
            n2786 = Concatenate Strings(w3582, ".duf" ("Substring")) -> (w3579:string)
            n2787 = String To Path(string=w3579) -> (path=w3583:path)
            n2788 = call <vilib>:"Read Characters From File.vi"("file path (dialog if empty)"=w3583, "start of read offset (chars.:0)"=60 ("start of read offset (chars.: 0)")) -> ("character string"=→"String Control 6":string)  [unwired: 4 in, 3 out]
          }
        }
        n2789 = case shown="True" "OPEN 4" {
          frame False {
          }
          frame True {
            (unwired) 0  # existing file
            w3604 = "Choose a datalog file to open"  # prompt
            n2790 = local write "OPEN 4"(FALSE ("OPEN 1")) -> ()
            n2791 = String To Path(string="C:\\LAB-IQ\\Data\\") -> (path=w3589:path)
            n2792 = File Dialog(6:"*.dgf" ("pattern"), 7:w3604, 11:w3589) -> (0:w3587:errorcluster, 3:w3595:path)  [unwired: 4 in, 2 out]
            n2793 = Unbundle(w3587) -> ()  [unwired: 3 out]
            n2794 = Strip Path(path=w3595) -> (name=w3593:string)  [unwired: 1 out]
            n2795 = Path To String(path=w3595) -> (string=w3590:string)
            "string1 4" <- w3590
            n2796 = Match Pattern(string=w3593, regular expression=".dgf") -> (before substring=→"String Control 7":string)  [unwired: 1 in, 3 out]
            n2797 = Match Pattern(string=w3590, regular expression=".dgf" ("substring (\"\")")) -> (before substring=w3600:string)  [unwired: 1 in, 3 out]
            n2798 = Concatenate Strings(w3600, ".duf" ("Substring")) -> (w3597:string)
            n2799 = String To Path(string=w3597) -> (path=w3601:path)
            n2800 = call <vilib>:"Read Characters From File.vi"("file path (dialog if empty)"=w3601, "start of read offset (chars.:0)"=60 ("start of read offset (chars.: 0)")) -> ("character string"=→"String Control 8":string)  [unwired: 4 in, 3 out]
          }
        }
      }
      frame "About" {
        # "Elapsed time\ncof\nstroke\nmean pos\nTemp\nHumidity"
        n2801 = disable-structure shown="Disabled" {
          frame Disabled {
            n2802 = case shown="True" "Export" {
              frame False {
              }
              frame True {
                w3626 = "                                      " ("string")
                w3628 = "\r"
                (unwired) i16 6 ("width (-)")
                w3705 = "\r"
                w3637 = "\r"
                n2803 = local write "Export"(FALSE ("Export")) -> ()
                n2804 = local read "String 29"() -> (w3674:string)
                n2805 = local read "String 34"() -> (w3662:string)
                n2806 = local read "String 35"() -> (w3657:string)
                n2807 = local read "String 37"() -> (w3653:string)
                n2808 = local read "String 36"() -> (w3650:string)
                n2809 = local read "String 38"() -> (w3647:string)
                n2810 = local read "String 39"() -> (w3644:string)
                n2811 = Match Pattern(string=w3674, regular expression=".dwm") -> (before substring=w3670:string)  [unwired: 1 in, 3 out]
                "before substring" <- w3670
                n2812 = local read "S 38"() -> (w3665:string)
                n2813 = local read "S 39"() -> (w3658:string)
                n2814 = local read "Temperature before test 2"() -> (w3694:dbl)
                n2815 = local read "Temperature after test 2"() -> (w3699:dbl)
                n2816 = local read "Humidity before test 2"() -> (w3680:dbl)
                n2817 = local read "Humidity after test 2"() -> (w3695:dbl)
                n2818 = local read "MWSD 2"() -> (w3691:dbl)
                n2819 = local read "WS1.4 2"() -> (w3707:dbl)
                n2820 = local read "HCF 2"() -> (w3703:dbl)
                n2821 = local read "AVP 2"() -> (w3692:dbl)
                n2822 = Concatenate Strings("1," ("string"), w3665) -> (w3664:string)
                n2823 = Concatenate Strings("2," ("string"), w3662) -> (w3661:string)
                n2824 = Concatenate Strings("3," ("string"), w3658) -> (w3660:string)
                n2825 = Concatenate Strings("4," ("string"), w3657) -> (w3656:string)
                n2826 = Concatenate Strings("5," ("string"), w3653) -> (w3654:string)
                n2827 = Concatenate Strings("6," ("string"), w3650) -> (w3651:string)
                n2828 = Concatenate Strings("7," ("string"), w3647) -> (w3648:string)
                n2829 = Concatenate Strings("8," ("string"), w3644) -> (w3645:string)
                n2830 = local read "Sample ID"() -> (w3712:string)
                n2831 = case shown="\"xlx\"" "Select File Type" {
                  tunnel: w3670 -> [w3715 w3717 w3719]
                  tunnel: [w3713 w3718 w3720] -> w3669
                  frame "xlx" {
                    n2832 = Concatenate Strings(w3715, ".xls" ("string")) -> (w3713:string)
                  }
                  frame "csv" {
                    n2833 = Concatenate Strings(w3717, ".csv" ("string")) -> (w3718:string)
                  }
                  frame "txt" {
                    n2834 = Concatenate Strings(w3719, ".txt" ("string")) -> (w3720:string)
                  }
                }
                n2835 = local read "Test Date"() -> (w3711:string)
                n2836 = local read "String 45"() -> (w3625:string)
                n2837 = local read "String 31"() -> (w3710:string)
                n2838 = local read "String 32"() -> (w3709:string)
                n2839 = local read "TITTLE"() -> (w3633:string)
                n2840 = Number To Fractional String(number=w3680, width (-)=i16 6, precision (6)=i16 2) -> (F-format string=w3679:string)  [unwired: 1 in]
                n2841 = Number To Fractional String(number=w3694, width (-)=i16 6, precision (6)=i16 2) -> (F-format string=w3700:string)  [unwired: 1 in]
                n2842 = Number To Fractional String(number=w3695, width (-)=i16 6, precision (6)=i16 2) -> (F-format string=w3693:string)  [unwired: 1 in]
                n2843 = Number To Fractional String(number=w3699, width (-)=i16 6, precision (6)=i16 2) -> (F-format string=w3698:string)  [unwired: 1 in]
                n2844 = Number To Fractional String(number=w3691, width (-)=i16 6, precision (6)=i16 2) -> (F-format string=w3689:string)  [unwired: 1 in]
                n2845 = Number To Fractional String(number=w3692, width (-)=i16 6, precision (6)=i16 2) -> (F-format string=w3690:string)  [unwired: 1 in]
                n2846 = Number To Fractional String(number=w3703, width (-)=i16 6, precision (6)=i16 2) -> (F-format string=w3704:string)  [unwired: 1 in]
                n2847 = Number To Fractional String(number=w3707, precision (6)=i16 2) -> (F-format string=w3708:string)  [unwired: 2 in]
                n2848 = local read "s.NO"() -> (w3627:string)
                n2849 = Concatenate Strings("=" ("string"), w3633) -> (w3632:string)
                n2850 = Concatenate Strings("S.No," ("string"), "                                       Parameters" ("string")) -> (w3638:string)
                n2851 = Concatenate Strings(w3705, w3664, w3679, w3705, w3661, w3700, w3705, w3660, w3693, w3705, w3656, w3698, w3705, w3654, w3689, w3705, w3651, w3690, w3705, w3648, w3704, w3705, w3645, w3708) -> (w3667:string)
                n2852 = Concatenate Strings(w3637, "," ("string"), w3625, w3627, w3626, w3709, w3712, w3626, w3710, w3711, w3637) -> (w3635:string)
                n2853 = local read "Tested by"() -> (w3641:string)
                n2854 = local read "String 33"() -> (w3642:string)
                n2855 = Concatenate Strings("," ("string"), "                                                                             " ("string")) -> (w3630:string)
                n2856 = Concatenate Strings(w3632, w3628, w3635, w3628, w3638, w3667, w3628, w3630, w3642, w3641) -> (→"export":string)
                n2857 = String To Path(string=w3669) -> (path=w3676:path)
                n2858 = local read "export"() -> (w3671:string)
                n2859 = call <vilib>:"Write Characters To File.vi"("append to file? (new file:F)"=FALSE, "character string"=w3671, "file path (dialog if empty)"=w3676) -> ()  [unwired: 2 in, 1 out]
              }
            }
          }
          frame Enabled {
          }
        }
        n2860 = case shown="True" "OK Button 17" {
          frame False {
          }
          frame True {
            (unwired) 0  # existing file
            w3929 = "Choose a datalog file to open"  # prompt
            n2861 = local write "OK Button 17"(FALSE ("OK Button 17")) -> ()
            n2862 = local read "String"() -> (w3924:string)
            n2863 = String To Path(string=w3924) -> (path=w3925:path)
            n2864 = File Dialog(6:"*.duf" ("pattern"), 7:w3929, 11:w3925) -> (0:w3916:errorcluster, 3:w3935:path)  [unwired: 4 in, 2 out]
            n2865 = Unbundle(w3916) -> ()  [unwired: 3 out]
            n2866 = Open/Create/Replace File "Open File"(file path (use dialog)=w3935) -> (refnum out=w3927:refnum<file>)  [unwired: 5 in, 2 out]
            n2867 = Strip Path(path=w3935) -> (name=w3933:string)  [unwired: 1 out]
            n2868 = Path To String(path=w3935) -> (string=w3918:string)
            n2869 = while {
              tunnel: w3927 -> [w3939]
              i -> [w3936]
              stop <- w3937 continue-if-true
              (unwired) TRUE ("line mode (F)")
              n2870 = Read from Text File "Read File"(file (use dialog)=w3939) -> (text=w3938:string)  [unwired: 3 in, 3 out]
              n2871 = local write "Numeric 16"(w3936) -> ()
              n2872 = String Length(string=w3938) -> (length=w3941:i32)
              n2873 = Greater?(x=w3941, y=1) -> (0:w3937:bool)
            }
            n2874 = local write "String 29"(w3918) -> ()
            n2875 = Search and Replace String(input string=w3918, search string=".duf", replace string=".dgf" ("replace string (\"\")")) -> (result string=→"String Indicator 4":string)  [unwired: 5 in, 3 out]
            n2876 = Match Pattern(string=w3933, regular expression=".dwm") -> (before substring=w3917:string)  [unwired: 1 in, 3 out]
            "String Indicator" <- w3917
            n2877 = Match Pattern(string=w3918, regular expression=".dwm" ("substring (\"\")")) -> (before substring=w3919:string)  [unwired: 1 in, 3 out]
            "String Indicator 3" <- w3919
            n2878 = local write "TITTLE 2"(w3917) -> ()
            n2879 = String To Path(string=w3919) -> (path=w3926:path)
            "path" <- w3926
            n2880 = call <vilib>:"Read Characters From File.vi"("file path (dialog if empty)"=w3926, "start of read offset (chars.:0)"=60 ("start of read offset (chars.: 0)")) -> ("character string"=→"String Indicator 2":string)  [unwired: 4 in, 3 out]
          }
        }
        n2881 = call <vilib>:"Query Available Printers.vi"() -> ("system configured printers"=w3618:string[])  [unwired: 9 in, 2 out]
        "System Configured Printers 2" <- w3618
        n2882 = local read "OK Button 16"() -> (w3615:bool)
        n2883 = case shown="True" "OK Button 16" {
          frame False {
          }
          frame True {
            n2884 = stacked-sequence {
              frame #0 {
                n2885 = local read "Numeric 16"() -> (w3943:i32)
                n2886 = local write "Numeric 10"(w3943) -> ()
              }
              frame #1 {
                n2887 = local read "String 29"() -> (w3946:string)
                n2888 = String To Path(string=w3946) -> (path=w3945:path)
                n2889 = Open/Create/Replace File "Open File"(file path (use dialog)=w3945) -> (refnum out=w3947:refnum<file>)  [unwired: 5 in, 2 out]
                n2890 = for {
                  N: 16 -> [_]
                  tunnel: w3947 -> [w3954]
                  i -> [w3950]
                  (unwired) TRUE ("line mode (F)")
                  n2891 = Read from Text File "Read File"(file (use dialog)=w3954) -> (text=w3948:string)  [unwired: 3 in, 3 out]
                  n2892 = Match Pattern(string=w3948, regular expression="(") -> (after substring=w3953:string)  [unwired: 1 in, 3 out]
                  n2893 = Match Pattern(string=w3953, regular expression=")") -> (before substring=w3949:string)  [unwired: 1 in, 3 out]
                  n2894 = case shown="1" w3950 {
